vi "GlobalWhereAmI.vi"() -> ()   [LabVIEW 2010]
panel:
  out "WhereAmI?":T1
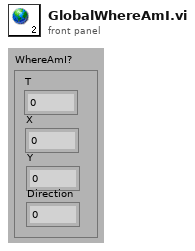
[diagram p1: front panel]
types:
  T1 = cluster{"T":dbl, "X":dbl, "Y":dbl, "Direction":dbl}
diagram:
